vi "Create ESPEC Tag.vi"(8 "error in (no error)":errorcluster, 11 "CVT Tags to Create":T1) -> (0 "error out":errorcluster, 3 "CVT Tags to Create 2":T1)   [LabVIEW 2021, in "CVT.lvlib"]
uses:
  CVT.lvlib
  <vilib>/NI/Current Value Table/Type Defs/File Format.ctl
  <vilib>/NI/Current Value Table/Type Defs/Single Tag.ctl
  <vilib>/NI/Current Value Table/Type Defs/Data Types.ctl
  <vilib>/NI/Current Value Table/Type Defs/Tag Grouping set.ctl
  <vilib>/NI/Current Value Table/Current Value Table.lvlib
panel:
  out "Humidity Data":T5
  out "Temp Data":T6
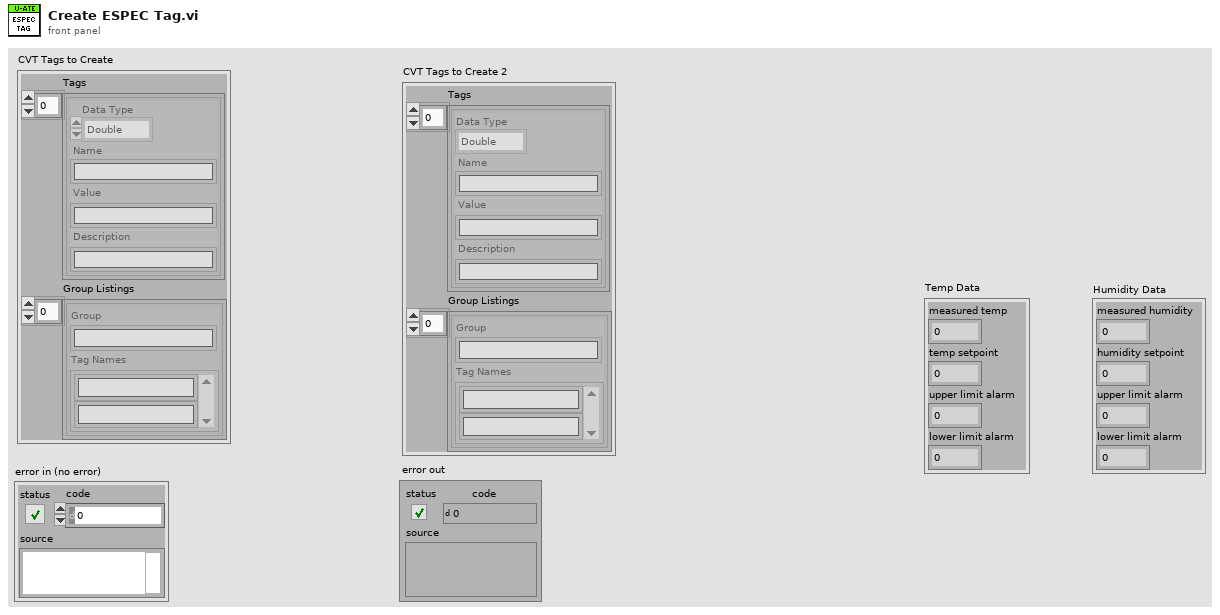
[diagram p1: front panel]
types:
  T1 = typedef "Current Value Table.lvlib/File Format.ctl" = cluster{"Tags":T2[], "Group Listings":T4[]}
  T2 = typedef "Current Value Table.lvlib/Single Tag.ctl" = cluster{"Data Type":T3, "Name":string, "Value":string, "Description":string}
  T3 = typedef "Current Value Table.lvlib/Data Types.ctl" = enum16{"Double", "Single", "I64", "I32", "I16", "I8", "U64", "U32", "U16", "U8", "String", "Boolean", "Array of U8", "Array of U16", "Array of U32", "Array of U64", "Array of I64", "Array of I32", "Array of I16", "Array of I8", "Array of Double", "Array of Single", "Array of Boolean", "Array of String"}
  T4 = typedef "Current Value Table.lvlib/Tag Grouping set.ctl" = cluster{"Group":string, "Tag Names":string[]}
  T5 = cluster{"measured humidity":dbl, "humidity setpoint":dbl, "upper limit alarm":dbl, "lower limit alarm":dbl}
  T6 = cluster{"measured temp":dbl, "temp setpoint":dbl, "upper limit alarm":dbl, "lower limit alarm":dbl}
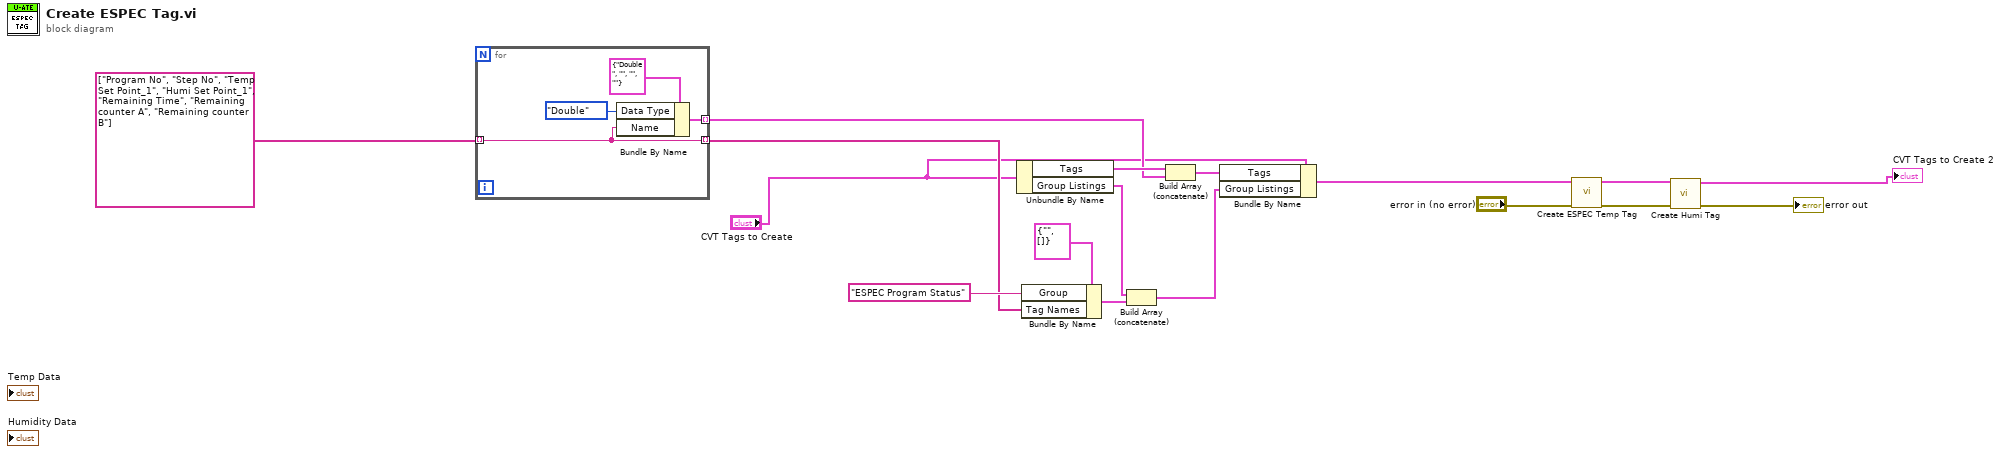
[diagram p0: block diagram]
diagram:
  n1 = for {
    tunnel: string[] ["Program No", "Step No", "Temp Set Point_1", "Humi Set Point_1", "Remaining Time", "Remaining counter A", "Remaining counter B"] -> [w20] mode=indexing
    tunnel: [w21] -> w16 mode=indexing
    tunnel: [w20] -> w13 mode=indexing
    n2 = Bundle By Name(cluster=T2 {"Data Type"=enum."Double", "Name"="", "Value"="", "Description"=""} ("Tag"), "Data Type"=Data_Types."Double", "Name"=w20) -> (w21:T2)
  }
  n3 = Unbundle By Name("CVT Tags to Create") -> ("Tags"=w17:T2[], "Group Listings"=w12:T4[])
  n4 = Bundle By Name(cluster=T4 {"Group"="", "Tag Names"=[]} ("Tag Grouping"), "Group"="ESPEC Program Status", "Tag Names"=w13) -> (w11:T4)
  n5 = Build Array (concatenate)(w12, w11) -> (w10:T4[])
  n6 = Build Array (concatenate)(w17, w16) -> (w15:T2[])
  n7 = Bundle By Name(cluster="CVT Tags to Create", "Tags"=w15, "Group Listings"=w10) -> (w8:T1)
  n8 = call "Create ESPEC Temp Tag.vi"("error in (no error)"="error in (no error)", "CVT Tags to Create"=w8) -> ("error out"=w5:errorcluster, "CVT Tags to Create 2"=w7:T1)  [unwired: 8 in]
  n9 = call "Create Humi Tag.vi"("error in (no error)"=w5, "CVT Tags to Create"=w7) -> ("error out"=→"error out":errorcluster, "CVT Tags to Create 2"=→"CVT Tags to Create 2":T1)  [unwired: 8 in]
